vi "Read Cfg Session.vi"(8 "error in (no error)":errorcluster, 11 "Instrument in":refnum<class "Instrument.lvclass">) -> (0 "error out":errorcluster, 2 "Session Handle":refnum<data-value>, 3 "Instrument out":refnum<class "Instrument.lvclass">)   [LabVIEW 2016, in "Instrument.lvclass"]
uses:
  Instrument.lvclass
  Session APIs/File Access/Config Data/Config Data.lvclass
  Instrument.lvclass/Instrument.ctl
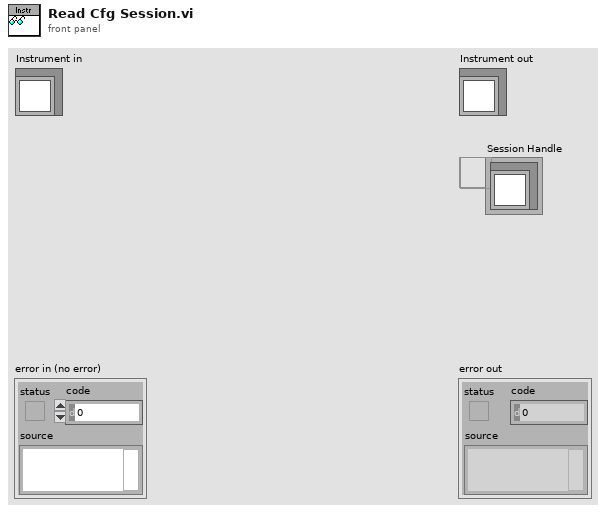
[diagram p1: front panel]
types:
  T1 = typedef "Session - Root.lvclass/Session Handle.ctl" = refnum<data-value>
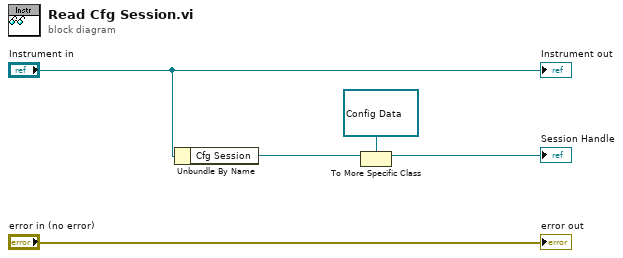
[diagram p0: block diagram]
diagram:
  n1 = Unbundle By Name("Instrument in") -> ("Cfg Session"=w3:T1)
  n2 = To More Specific Class(target class=refnum<data-value> refnum, reference=w3) -> (specific class reference=→"Session Handle":refnum<data-value>)  [unwired: 1 in, 1 out]
  "error out" <- "error in (no error)"
  "Instrument out" <- "Instrument in"
